vi "Create Aurora Resources.vi"() -> (3 "framework.resources":refnum<class "Register Configuration.lvclass">, 4 "config.resources":T7, 6 "sync.resources":T6, 8 "time.resources":T3, 10 "sfp 0.resources":T5, 14 "producer.resources":refnum<class "niInstr FIFO Register Bus v1 FPGA.lvclass">, 15 "sfp 1.resources":T4)   [LabVIEW 2016]
uses:
  <instrlib>/_niInstr/CLIP Adapters/v1/FPGA/AXI4-Lite/FXP32 Address - FXP32 Data/Public/CLIP Resources.ctl
  <instrlib>/_niInstr/CLIP Adapters/v1/FPGA/AXI4-Lite/FXP32 Address - FXP32 Data/niInstr AXI4-Lite - FXP32 Address - FXP32 Data v1 FPGA.lvclass
  <instrlib>/_niInstr/Instruction Framework/v1/FPGA/Top Level Bus/Register Configuration/Register Configuration.lvclass
  <instrlib>/_niInstr/FIFO Register Bus/v1/FPGA/niInstr FIFO Register Bus v1 FPGA.lvclass
  C:/Program Files (x86)/National Instruments/LabVIEW 2016/instr.lib/_niInstr/Instruction Framework/v1/FPGA/Interfaces/Instruction Producer/Instruction Producer.lvclass
  <instrlib>/_niInstr/CLIP Adapters/v1/FPGA/AXI4-Lite/Address Space Collection/niInstr AXI4-Lite Address Space Collection v1 FPGA.lvclass
  C:/Program Files (x86)/National Instruments/LabVIEW 2016/instr.lib/_niInstr/Instruction Framework/v1/FPGA/Interfaces/Address Space Collection/Address Space Collection.lvclass
  <instrlib>/niUsrpRio/Synchronization/v1/FPGA/Private/Resources.ctl
  <instrlib>/niUsrpRio/Synchronization/v1/FPGA/niUsrpRio Synchronization v1 FPGA.lvlib
  <instrlib>/_niInstr/CLIP Adapters/v1/FPGA/AXI4-Stream/Writer FXP64x1/niInstr AXI4-Stream Writer FXP64x1 v1 FPGA.lvclass
  <instrlib>/_niInstr/CLIP Adapters/v1/FPGA/AXI4-Stream/Reader FXP64x1/niInstr AXI4-Stream Reader FXP64x1 v1 FPGA.lvclass
  <instrlib>/niUsrpRio/Time/v1/FPGA/Private/Future Event Resources.ctl
  <instrlib>/niUsrpRio/Time/v1/FPGA/niUsrpRio Time v1 FPGA.lvlib
  <instrlib>/niUsrpRio/Time/v1/FPGA/Private/Time Resources.ctl
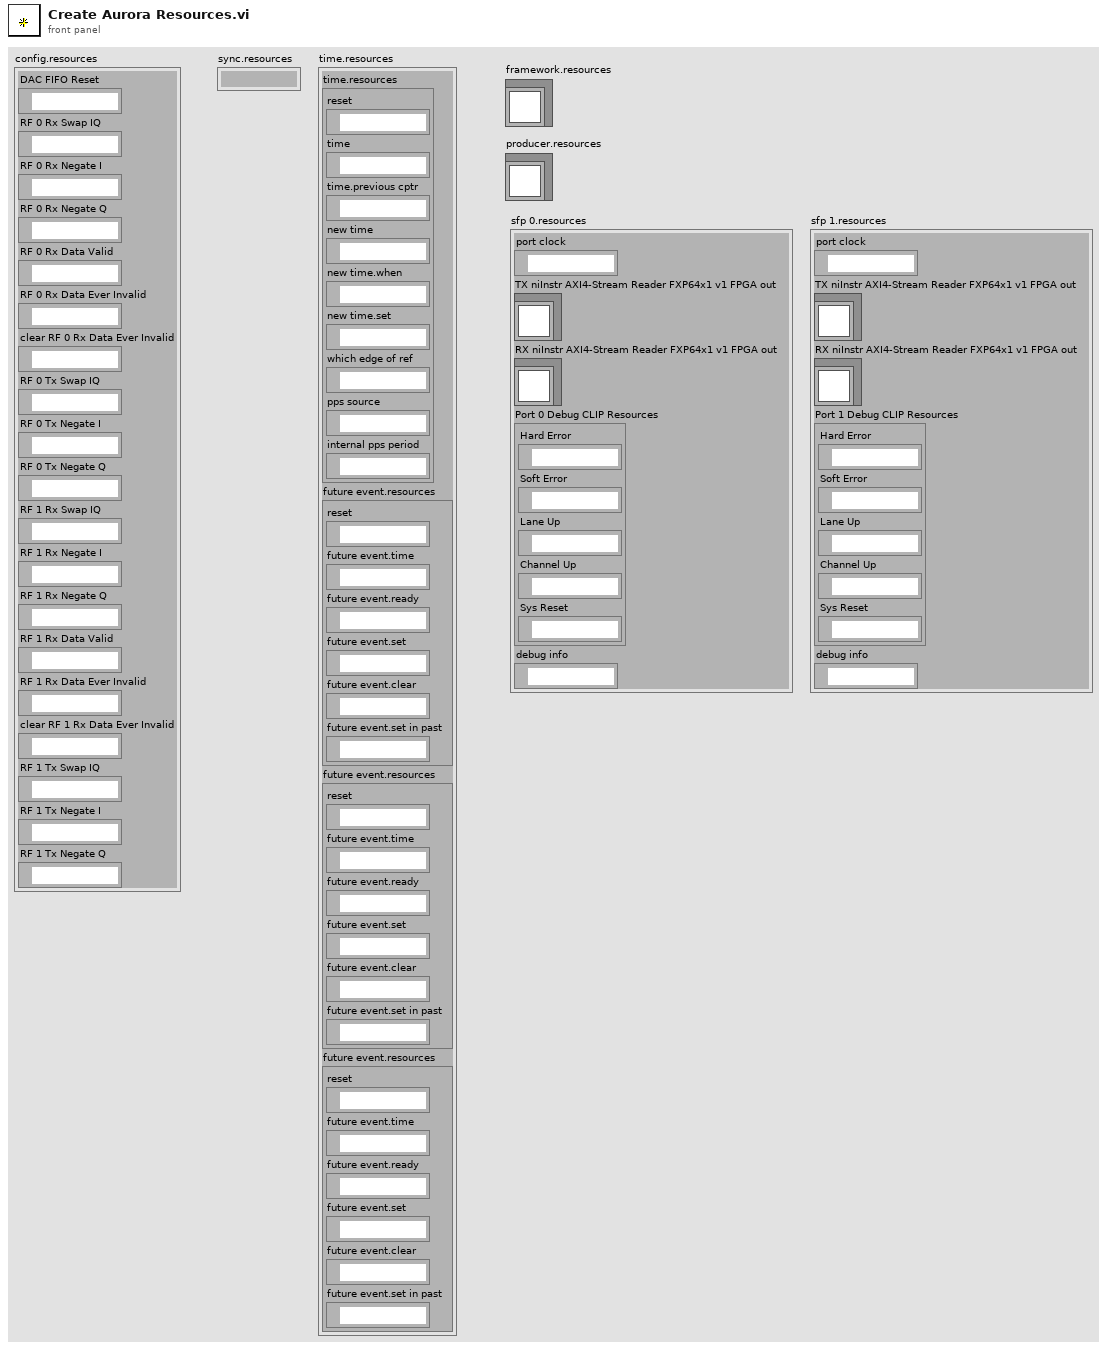
[diagram p1: front panel]
types:
  T1 = typedef "niUsrpRio Time v1 FPGA.lvlib/Time Resources.ctl" = cluster{"reset":refnum<k21>, "time":refnum<k21>, "time.previous cptr":refnum<k21>, "new time":refnum<k21>, "new time.when":refnum<k21>, "new time.set":refnum<k21>, "which edge of ref":refnum<k21>, "pps source":refnum<k21>, "internal pps period":refnum<k21>}
  T2 = typedef "niUsrpRio Time v1 FPGA.lvlib/Future Event Resources.ctl" = cluster{"reset":refnum<k21>, "future event.time":refnum<k21>, "future event.ready":refnum<k21>, "future event.set":refnum<k21>, "future event.clear":refnum<k21>, "future event.set in past":refnum<k21>}
  T3 = cluster{"time.resources":T1, "future event.resources":T2, "future event.resources":T2, "future event.resources":T2}
  T4 = cluster{"port clock":refnum<k21>, "TX niInstr AXI4-Stream Reader FXP64x1 v1 FPGA out":refnum<class "niInstr AXI4-Stream Writer FXP64x1 v1 FPGA.lvclass">, "RX niInstr AXI4-Stream Reader FXP64x1 v1 FPGA out":refnum<class "niInstr AXI4-Stream Reader FXP64x1 v1 FPGA.lvclass">, "Port 1 Debug CLIP Resources":cluster{"Hard Error":refnum<k21>, "Soft Error":refnum<k21>, "Lane Up":refnum<k21>, "Channel Up":refnum<k21>, "Sys Reset":refnum<k21>}, "debug info":refnum<k21>}
  T5 = cluster{"port clock":refnum<k21>, "TX niInstr AXI4-Stream Reader FXP64x1 v1 FPGA out":refnum<class "niInstr AXI4-Stream Writer FXP64x1 v1 FPGA.lvclass">, "RX niInstr AXI4-Stream Reader FXP64x1 v1 FPGA out":refnum<class "niInstr AXI4-Stream Reader FXP64x1 v1 FPGA.lvclass">, "Port 0 Debug CLIP Resources":cluster{"Hard Error":refnum<k21>, "Soft Error":refnum<k21>, "Lane Up":refnum<k21>, "Channel Up":refnum<k21>, "Sys Reset":refnum<k21>}, "debug info":refnum<k21>}
  T6 = typedef "niUsrpRio Synchronization v1 FPGA.lvlib/Resources.ctl" = cluster{"master":refnum<k21>, "meas.enable":refnum<k21>, "meas.ready":refnum<k21>, "meas.reset":refnum<k21>, "meas.arm":refnum<k21>, "meas.valid":refnum<k21>, "meas.value":refnum<k21>, "meas.oversample factor":refnum<k21>, "cptr":refnum<k21>, "cptr.adjust":refnum<k21>, "cptr.period":refnum<k21>}
  T7 = cluster{"DAC FIFO Reset":refnum<k21>, "RF 0 Rx Swap IQ":refnum<k21>, "RF 0 Rx Negate I":refnum<k21>, "RF 0 Rx Negate Q":refnum<k21>, "RF 0 Rx Data Valid":refnum<k21>, "RF 0 Rx Data Ever Invalid":refnum<k21>, "clear RF 0 Rx Data Ever Invalid":refnum<k21>, "RF 0 Tx Swap IQ":refnum<k21>, "RF 0 Tx Negate I":refnum<k21>, "RF 0 Tx Negate Q":refnum<k21>, "RF 1 Rx Swap IQ":refnum<k21>, "RF 1 Rx Negate I":refnum<k21>, "RF 1 Rx Negate Q":refnum<k21>, "RF 1 Rx Data Valid":refnum<k21>, "RF 1 Rx Data Ever Invalid":refnum<k21>, "clear RF 1 Rx Data Ever Invalid":refnum<k21>, "RF 1 Tx Swap IQ":refnum<k21>, "RF 1 Tx Negate I":refnum<k21>, "RF 1 Tx Negate Q":refnum<k21>}
  T8 = cluster{"Hard Error":refnum<k21>, "Soft Error":refnum<k21>, "Lane Up":refnum<k21>, "Channel Up":refnum<k21>, "Sys Reset":refnum<k21>}
  T9 = cluster{"m_axis_tvalid":refnum<k21>, "m_axis_tdata":refnum<k21>}
  T10 = cluster{"s_axis_tvalid":refnum<k21>, "s_axis_tdata":refnum<k21>, "s_axis_tready":refnum<k21>}
  T11 = typedef "niInstr AXI4-Lite - FXP32 Address - FXP32 Data v1 FPGA.lvclass/CLIP Resources.ctl" = cluster{"s_axi_araddr":refnum<k21>, "s_axi_arvalid":refnum<k21>, "s_axi_arready":refnum<k21>, "s_axi_rdata":refnum<k21>, "s_axi_rresp":refnum<k21>, "s_axi_rvalid":refnum<k21>, "s_axi_rready":refnum<k21>, "s_axi_awaddr":refnum<k21>, "s_axi_awvalid":refnum<k21>, "s_axi_awready":refnum<k21>, "s_axi_wdata":refnum<k21>, "s_axi_wstrb":refnum<k21>, "s_axi_wvalid":refnum<k21>, "s_axi_wready":refnum<k21>, "s_axi_bresp":refnum<k21>, "s_axi_bvalid":refnum<k21>, "s_axi_bready":refnum<k21>}
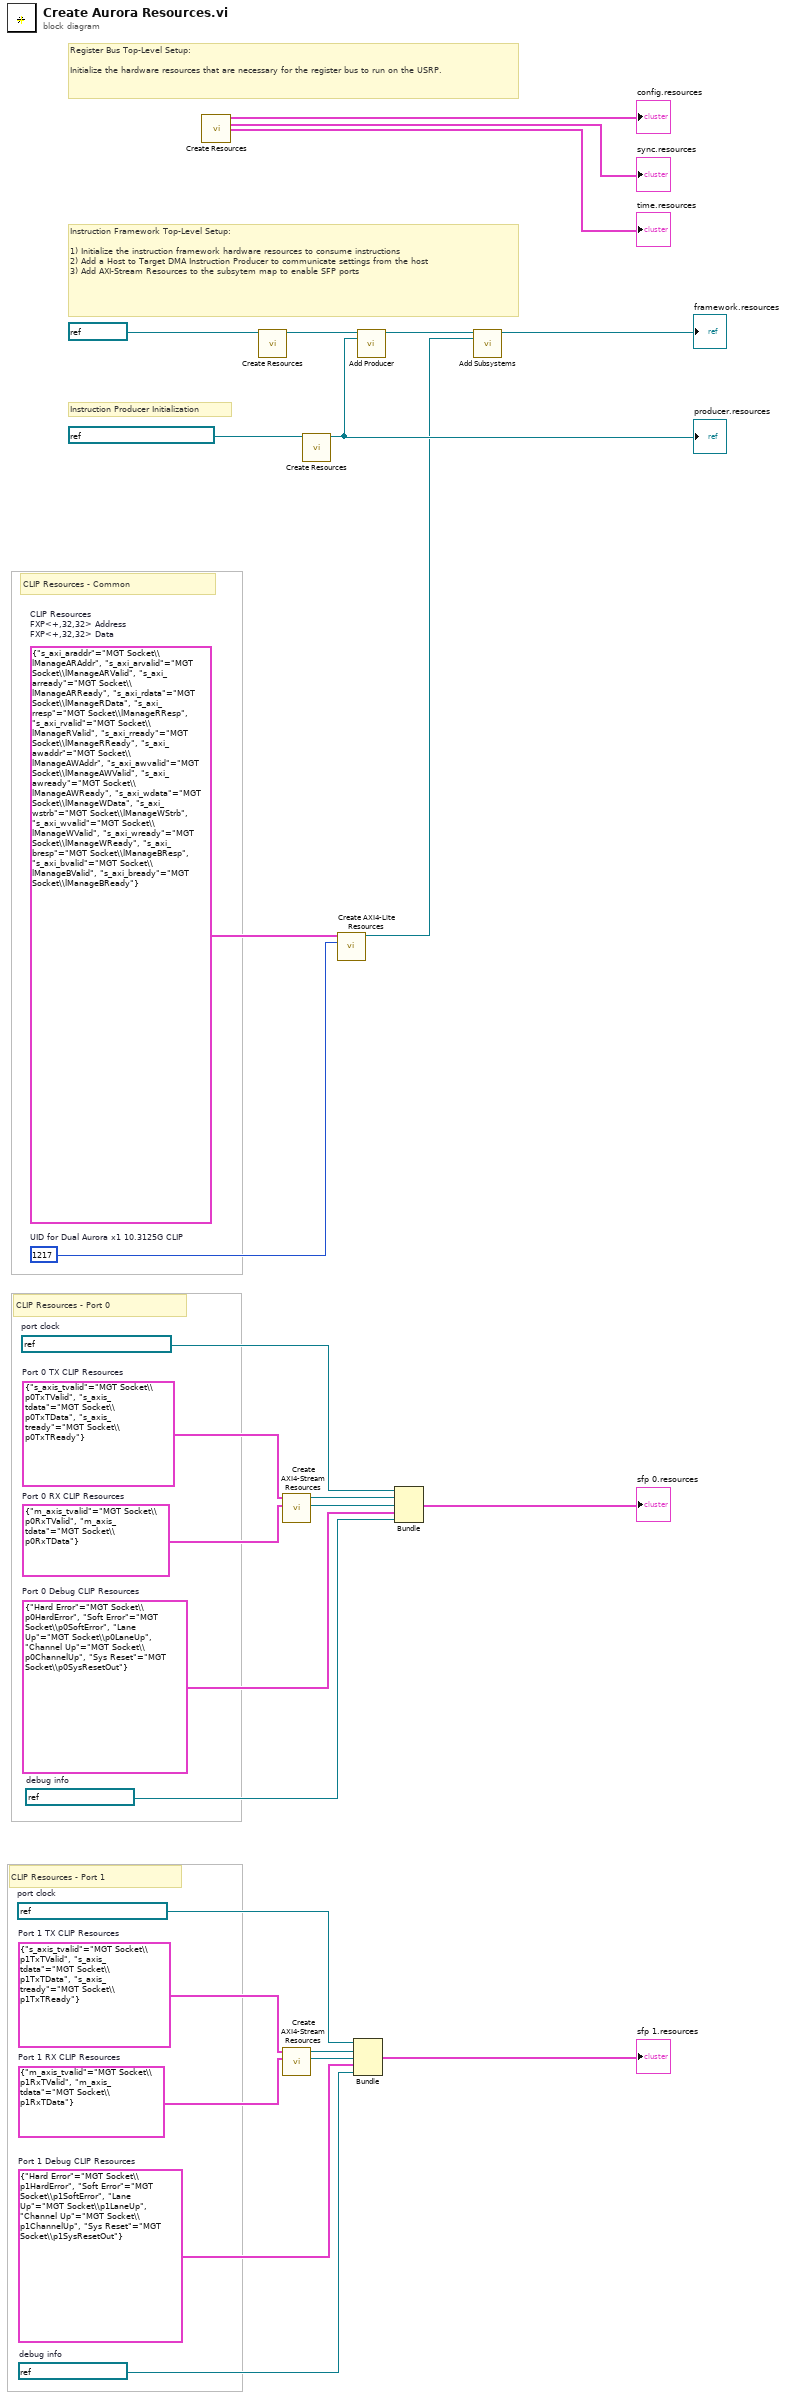
[diagram p0: block diagram]
diagram:
  w21 = refnum<k21> "port 1 debug info"  # debug info
  w6 = refnum<k21> "port 0 debug info"  # debug info
  w22 = T8 {"Hard Error"="MGT Socket\\p1HardError", "Soft Error"="MGT Socket\\p1SoftError", "Lane Up"="MGT Socket\\p1LaneUp", "Channel Up"="MGT Socket\\p1ChannelUp", "Sys Reset"="MGT Socket\\p1SysResetOut"}  # Port 1 Debug CLIP Resources
  w18 = T9 {"m_axis_tvalid"="MGT Socket\\p1RxTValid", "m_axis_tdata"="MGT Socket\\p1RxTData"}  # Port 1 RX CLIP Resources
  w17 = T10 {"s_axis_tvalid"="MGT Socket\\p1TxTValid", "s_axis_tdata"="MGT Socket\\p1TxTData", "s_axis_tready"="MGT Socket\\p1TxTReady"}  # Port 1 TX CLIP Resources
  w23 = refnum<k21> "MGT Socket\\Port1UserClk"  # port clock
  w5 = T8 {"Hard Error"="MGT Socket\\p0HardError", "Soft Error"="MGT Socket\\p0SoftError", "Lane Up"="MGT Socket\\p0LaneUp", "Channel Up"="MGT Socket\\p0ChannelUp", "Sys Reset"="MGT Socket\\p0SysResetOut"}  # Port 0 Debug CLIP Resources
  w19 = T9 {"m_axis_tvalid"="MGT Socket\\p0RxTValid", "m_axis_tdata"="MGT Socket\\p0RxTData"}  # Port 0 RX CLIP Resources
  w20 = T10 {"s_axis_tvalid"="MGT Socket\\p0TxTValid", "s_axis_tdata"="MGT Socket\\p0TxTData", "s_axis_tready"="MGT Socket\\p0TxTReady"}  # Port 0 TX CLIP Resources
  w2 = refnum<k21> "MGT Socket\\Port0UserClk"  # port clock
  w24 = u16 1217  # UID for Dual Aurora x1 10.3125G CLIP
  w25 = T11 {"s_axi_araddr"="MGT Socket\\lManageARAddr", "s_axi_arvalid"="MGT Socket\\lManageARValid", "s_axi_arready"="MGT Socket\\lManageARReady", "s_axi_rdata"="MGT Socket\\lManageRData", "s_axi_rresp"="MGT Socket\\lManageRResp", "s_axi_rvalid"="MGT Socket\\lManageRValid", "s_axi_rready"="MGT Socket\\lManageRReady", "s_axi_awaddr"="MGT Socket\\lManageAWAddr", "s_axi_awvalid"="MGT Socket\\lManageAWValid", "s_axi_awready"="MGT Socket\\lManageAWReady", "s_axi_wdata"="MGT Socket\\lManageWData", "s_axi_wstrb"="MGT Socket\\lManageWStrb", "s_axi_wvalid"="MGT Socket\\lManageWValid", "s_axi_wready"="MGT Socket\\lManageWReady", "s_axi_bresp"="MGT Socket\\lManageBResp", "s_axi_bvalid"="MGT Socket\\lManageBValid", "s_axi_bready"="MGT Socket\\lManageBReady"}  # CLIP Resources FXP<+,32,32> Address FXP<+,32,32> Data
  # "Instruction Producer Initialization"
  # "Instruction Framework Top-Level Setup: \n\n1) Initialize the instruction framework hardware resources to consume instructions\n2) Add a Host to Target DMA Instruction Producer to communicate settings from the host\n3) Add AXI-Stream Resources to the subsytem map to enable SFP ports"
  # "CLIP Resources - Port 1"
  # "CLIP Resources - Port 0"
  # "CLIP Resources - Common"
  # "Register Bus Top-Level Setup: \n\nInitialize the hardware resources that are necessary for the register bus to run on the USRP."
  n1 = call <instrlib>:"Create Resources.vi"() -> ("config.resources"=→"config.resources":T7, "sync.resources"=→"sync.resources":T6, "time.resources"=→"time.resources":T3)  [unwired: 13 in]
  n2 = call <instrlib>:"Create Resources.vi"("register clock"=refnum<k21> "50MHz" ("FPGA Clock")) -> ("register configuration"=w9:refnum<class "Register Configuration.lvclass">)  [unwired: 14 in]
  n3 = call "Create AXI4-Stream Resources.vi"("RX CLIP Resources"=w19, "TX CLIP Resources"=w20) -> ("RX niInstr AXI4-Stream Reader FXP64x1 v1 FPGA out"=w4:refnum<class "niInstr AXI4-Stream Reader FXP64x1 v1 FPGA.lvclass">, "TX niInstr AXI4-Stream Reader FXP64x1 v1 FPGA out"=w3:refnum<class "niInstr AXI4-Stream Writer FXP64x1 v1 FPGA.lvclass">)  [unwired: 8 in]
  n4 = call "Create AXI4-Stream Resources.vi"("RX CLIP Resources"=w18, "TX CLIP Resources"=w17) -> ("RX niInstr AXI4-Stream Reader FXP64x1 v1 FPGA out"=w15:refnum<class "niInstr AXI4-Stream Reader FXP64x1 v1 FPGA.lvclass">, "TX niInstr AXI4-Stream Reader FXP64x1 v1 FPGA out"=w16:refnum<class "niInstr AXI4-Stream Writer FXP64x1 v1 FPGA.lvclass">)  [unwired: 8 in]
  n5 = call <instrlib>:"Create Resources.vi"("instruction fifo"=refnum<k21> "reg.host instruction fifo 1" ("FIFO")) -> ("fifo register bus"=w13:refnum<class "niInstr FIFO Register Bus v1 FPGA.lvclass">)  [unwired: 14 in]
  "producer.resources" <- w13
  n6 = call "Create AXI4-Lite Resources.vi"("CLIP Resources\nFXP<+,32,32> Address\nFXP<+,32,32> Data"=w25, "UID for Dual Aurora x1 10.3125G CLIP"=w24) -> ("niInstr AXI4-Lite Address Space Collection v1 FPGA out"=w7:refnum<class "niInstr AXI4-Lite Address Space Collection v1 FPGA.lvclass">)  [unwired: 13 in]
  n7 = Bundle("port clock"=w23, "TX niInstr AXI4-Stream Reader FXP64x1 v1 FPGA out"=w16, "RX niInstr AXI4-Stream Reader FXP64x1 v1 FPGA out"=w15, "Port 1 Debug CLIP Resources"=w22, "debug info"=w21) -> (→"sfp 1.resources":T4)  [unwired: 1 in]
  n8 = call <instrlib>:"Add Producer.vi"("register configuration in"=w9, "instruction producer"=w13) -> ("register configuration out"=w10:refnum<class "Register Configuration.lvclass">)  [unwired: 13 in]
  n9 = Bundle("port clock"=w2, "TX niInstr AXI4-Stream Reader FXP64x1 v1 FPGA out"=w3, "RX niInstr AXI4-Stream Reader FXP64x1 v1 FPGA out"=w4, "Port 0 Debug CLIP Resources"=w5, "debug info"=w6) -> (→"sfp 0.resources":T5)  [unwired: 1 in]
  n10 = call <instrlib>:"Add Subsystems.vi"("register configuration in"=w10, "subsystems"=w7) -> ("register configuration out"=→"framework.resources":refnum<class "Register Configuration.lvclass">)  [unwired: 13 in]
